vi "Find Differential Pair.vi"(10 "Chainnel Index":i32, 11 "Channel Definitions":cluster{"Channel":string, "Source":string}[](array[cluster])) -> (1 "Pair Found?":bool, 2 "Channel Pair Index":i32)   [LabVIEW 2020, in "Routing and Faulting System Explorer.lvlib"]
uses:
  Routing and Faulting System Explorer.lvlib
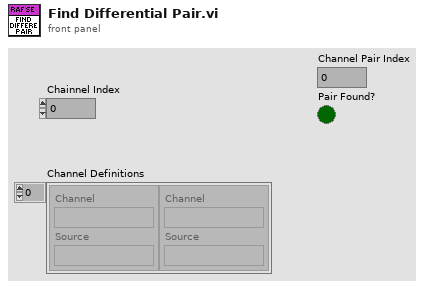
[diagram p1: front panel]
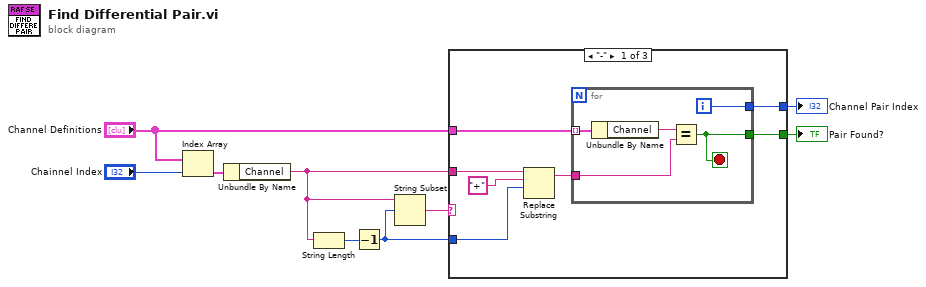
[diagram p0: block diagram]
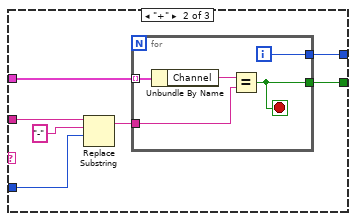
[diagram p2: hidden frame]
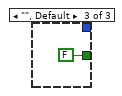
[diagram p3: hidden frame]
diagram:
  n1 = Index Array(array="Channel Definitions", index="Chainnel Index") -> (element=w5:cluster{"Channel":string, "Source":string})
  n2 = Unbundle By Name(w5) -> ("Channel"=w9:string)
  n3 = String Length(string=w9) -> (length=w6:i32)
  n4 = Decrement(x=w6) -> (x-1=w3:i32)
  n5 = String Subset(string=w9, offset (0)=w3) -> (substring=w7:string)  [unwired: 1 in]
  n6 = case shown="\"-\"" w7 {
    tunnel: "Channel Definitions" -> [w13 w25 _]
    tunnel: w9 -> [w16 w28 _]
    tunnel: w3 -> [w15 w27 _]
    tunnel: [w11 w23 _] -> w2
    tunnel: [w10 w22 FALSE] -> w1
    frame "-" {
      n7 = Replace Substring(3:w15, 4:"+" ("substring (\"\")"), 5:w16) -> (1:w12:string)  [unwired: 1 in, 1 out]
      n8 = for {
        tunnel: w13 -> [w21] mode=indexing
        tunnel: w12 -> [w19]
        tunnel: [w18] -> w10
        tunnel: [w17] -> w11
        i -> [w17]
        stop <- w18 stop-if-true
        n9 = Unbundle By Name(w21) -> ("Channel"=w20:string)
        n10 = Equal?(x=w20, y=w19) -> (x = y?=w18:bool)
      }
    }
    frame "+" {
      n11 = Replace Substring(3:w27, 4:"-" ("substring (\"\")"), 5:w28) -> (1:w24:string)  [unwired: 1 in, 1 out]
      n12 = for {
        tunnel: w25 -> [w33] mode=indexing
        tunnel: w24 -> [w31]
        tunnel: [w30] -> w22
        tunnel: [w29] -> w23
        i -> [w29]
        stop <- w30 stop-if-true
        n13 = Unbundle By Name(w33) -> ("Channel"=w32:string)
        n14 = Equal?(x=w32, y=w31) -> (x = y?=w30:bool)
      }
    }
    frame "", Default {
    }
  }
  "Channel Pair Index" <- w2
  "Pair Found?" <- w1
